vi "Process Messages.vi"(8 "error in (no error)":errorcluster, 11 "Mixer in":refnum<class "Mixer.lvclass">) -> (0 "error out":errorcluster, 3 "Mixer out":refnum<class "Mixer.lvclass">)   [LabVIEW 2019, in "Mixer.lvclass"]
uses:
  Mixer.lvclass
  Mixer.lvclass/Mixer.ctl
  Channel/Channel.lvclass
  Libraries/Messaging/Messaging.lvlib
  Libraries/Audio Processing/Audio Processing.lvlib
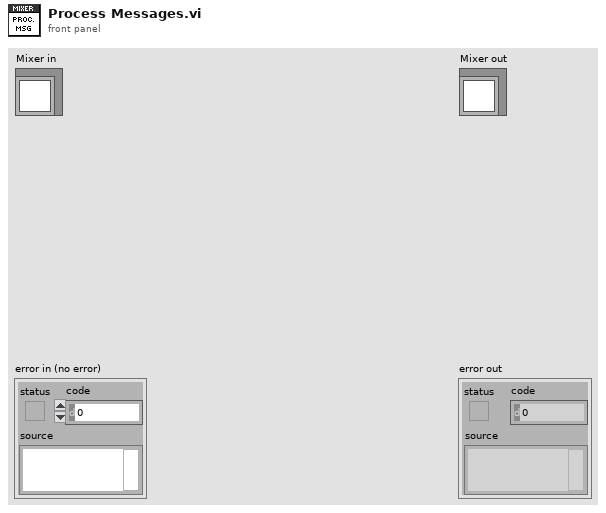
[diagram p1: front panel]
types:
  T1 = typedef "Messaging.lvlib/Message Cluster.ctl" = cluster{"Event":string, "Source":string, "Target":string, "Data":variant}
  T2 = typedef "Audio Processing.lvlib/Value Properties.ctl" = cluster{"Lower":dbl, "Upper":dbl}
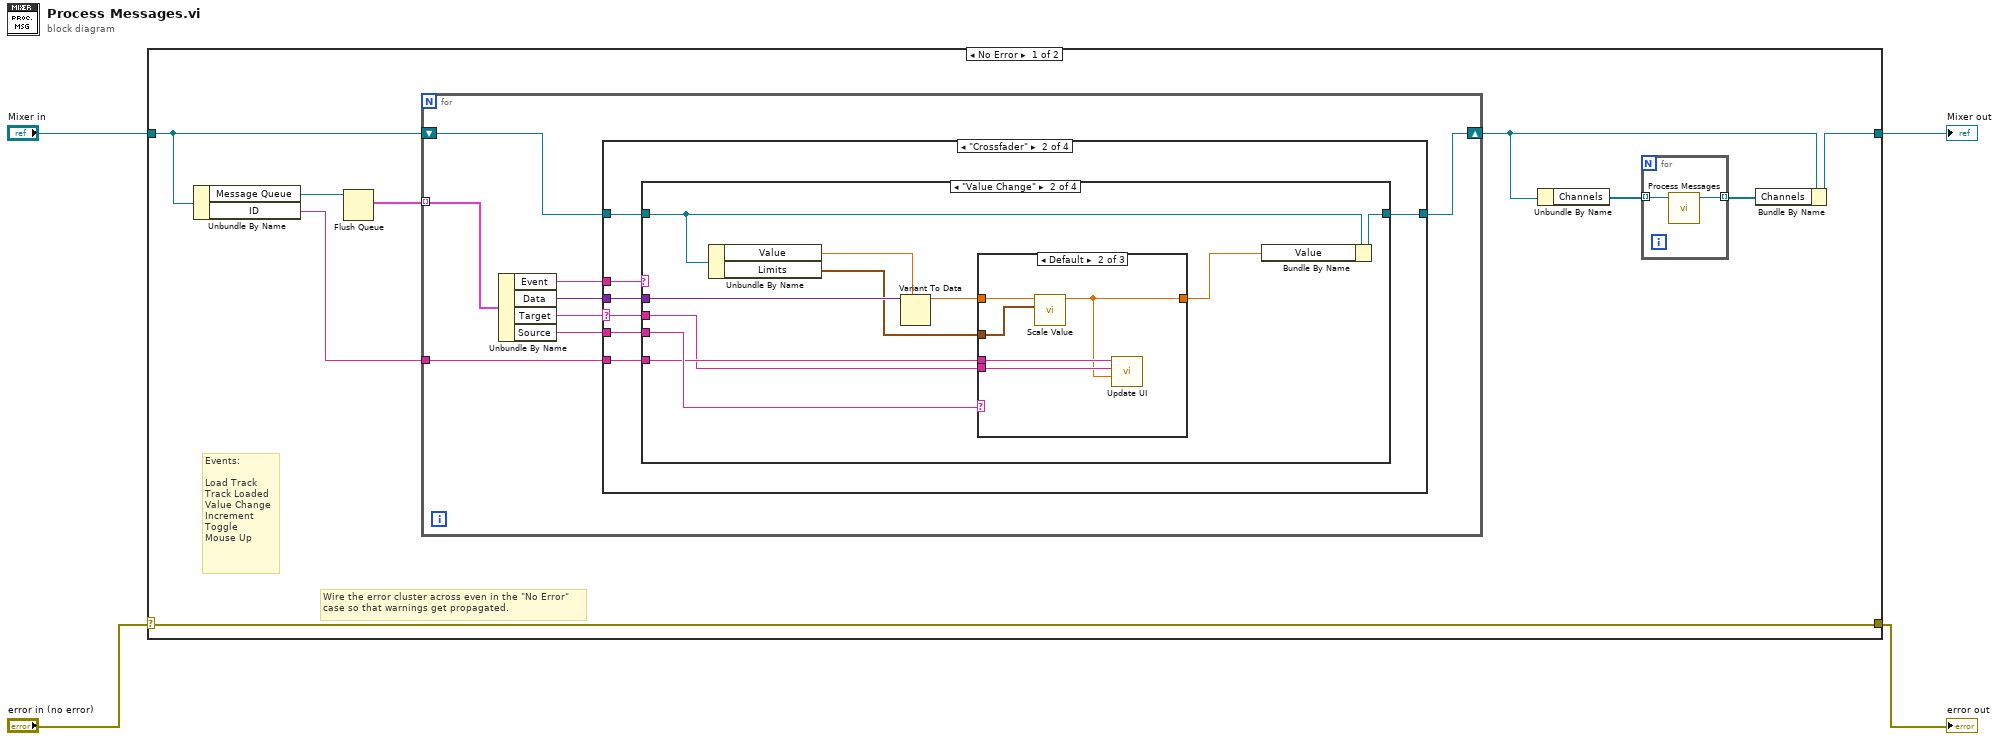
[diagram p0: block diagram]
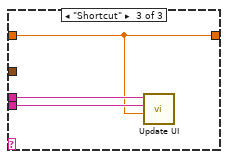
[diagram p5: hidden frame]
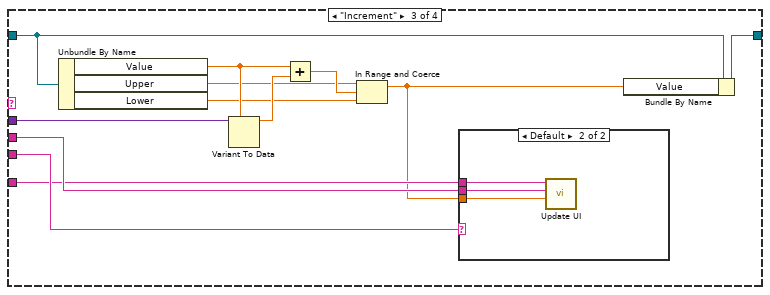
[diagram p6: hidden frame]
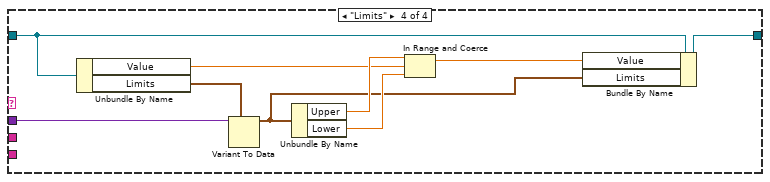
[diagram p8: hidden frame]
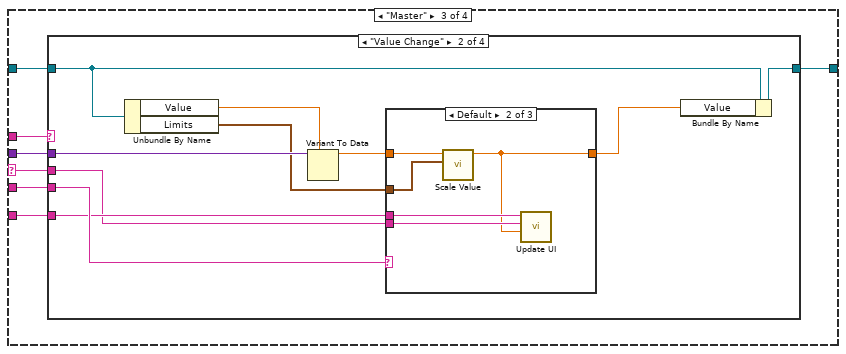
[diagram p9: hidden frame]
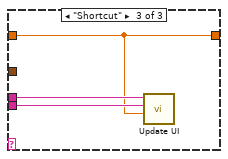
[diagram p12: hidden frame]
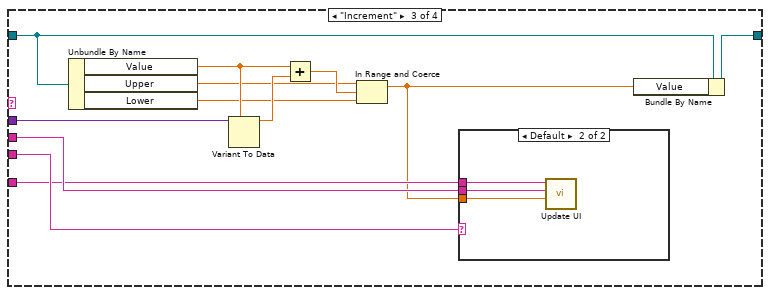
[diagram p13: hidden frame]
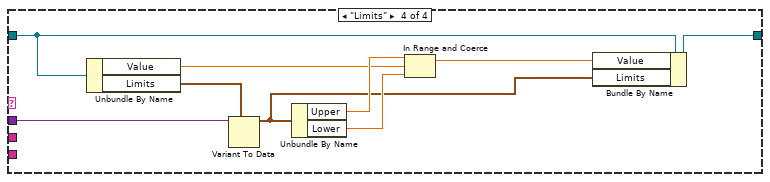
[diagram p15: hidden frame]
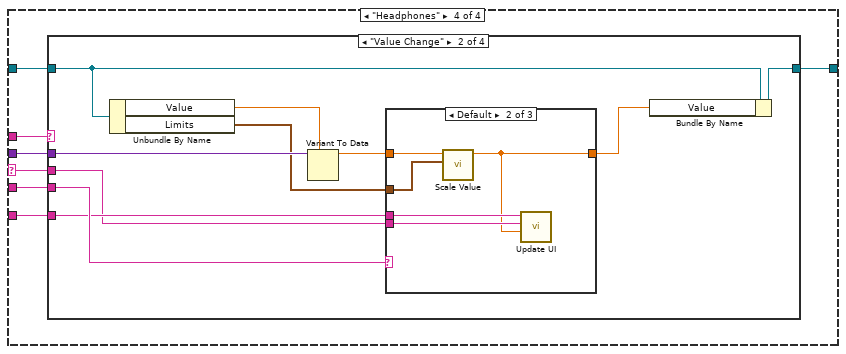
[diagram p16: hidden frame]
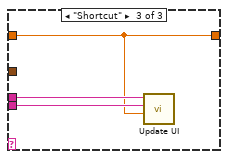
[diagram p19: hidden frame]
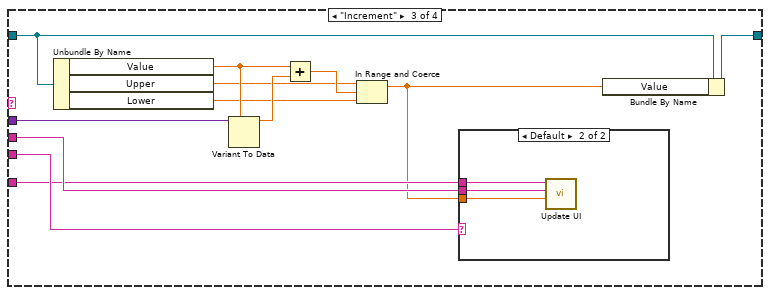
[diagram p20: hidden frame]
diagram:
  n1 = case shown="No Error" "error in (no error)" {
    selector: "error in (no error)" -> [w13 w179]
    tunnel: [w13 w179] -> w2
    tunnel: [w8 w178] -> w1
    tunnel: "Mixer in" -> [w12 w178]
    frame No Error {
      # "Events:\n\nLoad Track\nTrack Loaded\nValue Change\nIncrement\nToggle\nMouse Up"
      # "Wire the error cluster across even in the \"No Error\"\ncase so that warnings get propagated."
      n2 = Unbundle By Name(w12) -> ("Message Queue"=w7:refnum<queue>, "ID"=w5:string)
      n3 = Flush Queue(queue=w7) -> (remaining elements=w6:T1[])  [unwired: 1 in, 2 out]
      n4 = for {
        shift-right: [w22] -> w9
        shift-left: w12 -> [w23]
        tunnel: w6 -> [w21] mode=indexing
        tunnel: w5 -> [w16]
        n5 = Unbundle By Name(w21) -> ("Event"=w18:string, "Data"=w19:variant, "Target"=w20:string, "Source"=w17:string)
        n6 = case shown="\"Crossfader\"" w20 {
          selector: w20 -> [_ w26 w79 w130]
          tunnel: w23 -> [w24 w29 w82 w133]
          tunnel: [w24 w30 w76 w127] -> w22
          tunnel: w19 -> [_ w28 w80 w131]
          tunnel: w18 -> [_ w31 w81 w132]
          tunnel: w17 -> [_ w27 w78 w129]
          tunnel: w16 -> [_ w25 w77 w128]
          frame Default {
          }
          frame "Crossfader" {
            n7 = case shown="\"Value Change\"" w31 {
              tunnel: [w32 w39 w61 w73] -> w30
              tunnel: w29 -> [w32 w40 w62 w74]
              tunnel: w28 -> [_ w41 w63 w75]
              tunnel: w27 -> [_ w37 w60 _]
              tunnel: w26 -> [_ w35 w59 _]
              tunnel: w25 -> [_ w36 w58 _]
              frame Default {
              }
              frame "Value Change" {
                n8 = Unbundle By Name(w40) -> ("Value"=w42:dbl, "Limits"=w33:T2)
                n9 = Variant To Data(type=w42, Variant=w41) -> (data=w38:dbl)  [unwired: 1 in, 1 out]
                n10 = case shown="Default" w37 {
                  tunnel: w38 -> [w43 w46 w49]
                  tunnel: w35 -> [_ w48 w51]
                  tunnel: w36 -> [_ w47 w50]
                  tunnel: [w43 w44 w49] -> w34
                  tunnel: w33 -> [_ w45 _]
                  frame "UI" {
                  }
                  frame Default {
                    n11 = call "Scale Value.vi"("Limits"=w45, "Value"=w46) -> ("Scaled Value"=w44:dbl)  [unwired: 9 in]
                    n12 = call "Update UI.vi"("Data"=w44, "Target"=w48, "ID"=w47) -> ()  [unwired: 8 in, 1 out]
                  }
                  frame "Shortcut" {
                    n13 = call "Update UI.vi"("Data"=w49, "Target"=w51, "ID"=w50) -> ()  [unwired: 8 in, 1 out]
                  }
                }
                n14 = Bundle By Name(cluster=w40, "Value"=w34) -> (w39:refnum<class "Mixer.lvclass">)
              }
              frame "Increment" {
                n15 = Unbundle By Name(w62) -> ("Value"=w57:dbl, "Upper"=w54:dbl, "Lower"=w53:dbl)
                n16 = Variant To Data(type=w57, Variant=w63) -> (data=w56:dbl)  [unwired: 1 in, 1 out]
                n17 = Add(x=w57, y=w56) -> (x+y=w55:dbl)
                n18 = In Range and Coerce(upper limit=w54, x=w55, lower limit=w53) -> (coerced(x)=w52:dbl)  [unwired: 1 out]
                n19 = case shown="Default" w60 {
                  tunnel: w52 -> [_ w66]
                  tunnel: w59 -> [_ w65]
                  tunnel: w58 -> [_ w64]
                  frame "UI" {
                  }
                  frame Default {
                    n20 = call "Update UI.vi"("Data"=w66, "Target"=w65, "ID"=w64) -> ()  [unwired: 8 in, 1 out]
                  }
                }
                n21 = Bundle By Name(cluster=w62, "Value"=w52) -> (w61:refnum<class "Mixer.lvclass">)
              }
              frame "Limits" {
                n22 = Unbundle By Name(w74) -> ("Value"=w69:dbl, "Limits"=w67:T2)
                n23 = Variant To Data(type=w67, Variant=w75) -> (data=w68:T2)  [unwired: 1 in, 1 out]
                n24 = Unbundle By Name(w68) -> ("Upper"=w71:dbl, "Lower"=w70:dbl)
                n25 = In Range and Coerce(upper limit=w71, x=w69, lower limit=w70) -> (coerced(x)=w72:dbl)  [unwired: 1 out]
                n26 = Bundle By Name(cluster=w74, "Value"=w72, "Limits"=w68) -> (w73:refnum<class "Mixer.lvclass">)
              }
            }
          }
          frame "Master" {
            n27 = case shown="\"Value Change\"" w81 {
              tunnel: [w83 w90 w112 w124] -> w76
              tunnel: w82 -> [w83 w91 w113 w125]
              tunnel: w80 -> [_ w92 w114 w126]
              tunnel: w78 -> [_ w88 w111 _]
              tunnel: w79 -> [_ w86 w110 _]
              tunnel: w77 -> [_ w87 w109 _]
              frame Default {
              }
              frame "Value Change" {
                n28 = Unbundle By Name(w91) -> ("Value"=w93:dbl, "Limits"=w84:T2)
                n29 = Variant To Data(type=w93, Variant=w92) -> (data=w89:dbl)  [unwired: 1 in, 1 out]
                n30 = case shown="Default" w88 {
                  tunnel: w89 -> [w94 w97 w100]
                  tunnel: w86 -> [_ w99 w102]
                  tunnel: w87 -> [_ w98 w101]
                  tunnel: [w94 w95 w100] -> w85
                  tunnel: w84 -> [_ w96 _]
                  frame "UI" {
                  }
                  frame Default {
                    n31 = call "Scale Value.vi"("Limits"=w96, "Value"=w97) -> ("Scaled Value"=w95:dbl)  [unwired: 9 in]
                    n32 = call "Update UI.vi"("Data"=w95, "Target"=w99, "ID"=w98) -> ()  [unwired: 8 in, 1 out]
                  }
                  frame "Shortcut" {
                    n33 = call "Update UI.vi"("Data"=w100, "Target"=w102, "ID"=w101) -> ()  [unwired: 8 in, 1 out]
                  }
                }
                n34 = Bundle By Name(cluster=w91, "Value"=w85) -> (w90:refnum<class "Mixer.lvclass">)
              }
              frame "Increment" {
                n35 = Unbundle By Name(w113) -> ("Value"=w108:dbl, "Upper"=w105:dbl, "Lower"=w104:dbl)
                n36 = Variant To Data(type=w108, Variant=w114) -> (data=w107:dbl)  [unwired: 1 in, 1 out]
                n37 = Add(x=w108, y=w107) -> (x+y=w106:dbl)
                n38 = In Range and Coerce(upper limit=w105, x=w106, lower limit=w104) -> (coerced(x)=w103:dbl)  [unwired: 1 out]
                n39 = case shown="Default" w111 {
                  tunnel: w103 -> [_ w117]
                  tunnel: w110 -> [_ w116]
                  tunnel: w109 -> [_ w115]
                  frame "UI" {
                  }
                  frame Default {
                    n40 = call "Update UI.vi"("Data"=w117, "Target"=w116, "ID"=w115) -> ()  [unwired: 8 in, 1 out]
                  }
                }
                n41 = Bundle By Name(cluster=w113, "Value"=w103) -> (w112:refnum<class "Mixer.lvclass">)
              }
              frame "Limits" {
                n42 = Unbundle By Name(w125) -> ("Value"=w120:dbl, "Limits"=w118:T2)
                n43 = Variant To Data(type=w118, Variant=w126) -> (data=w119:T2)  [unwired: 1 in, 1 out]
                n44 = Unbundle By Name(w119) -> ("Upper"=w122:dbl, "Lower"=w121:dbl)
                n45 = In Range and Coerce(upper limit=w122, x=w120, lower limit=w121) -> (coerced(x)=w123:dbl)  [unwired: 1 out]
                n46 = Bundle By Name(cluster=w125, "Value"=w123, "Limits"=w119) -> (w124:refnum<class "Mixer.lvclass">)
              }
            }
          }
          frame "Headphones" {
            n47 = case shown="\"Value Change\"" w132 {
              tunnel: [w134 w141 w163 w175] -> w127
              tunnel: w133 -> [w134 w142 w164 w176]
              tunnel: w131 -> [_ w143 w165 w177]
              tunnel: w129 -> [_ w139 w162 _]
              tunnel: w130 -> [_ w137 w161 _]
              tunnel: w128 -> [_ w138 w160 _]
              frame Default {
              }
              frame "Value Change" {
                n48 = Unbundle By Name(w142) -> ("Value"=w144:dbl, "Limits"=w135:T2)
                n49 = Variant To Data(type=w144, Variant=w143) -> (data=w140:dbl)  [unwired: 1 in, 1 out]
                n50 = case shown="Default" w139 {
                  tunnel: w140 -> [w145 w148 w151]
                  tunnel: w137 -> [_ w150 w153]
                  tunnel: w138 -> [_ w149 w152]
                  tunnel: [w145 w146 w151] -> w136
                  tunnel: w135 -> [_ w147 _]
                  frame "UI" {
                  }
                  frame Default {
                    n51 = call "Scale Value.vi"("Limits"=w147, "Value"=w148) -> ("Scaled Value"=w146:dbl)  [unwired: 9 in]
                    n52 = call "Update UI.vi"("Data"=w146, "Target"=w150, "ID"=w149) -> ()  [unwired: 8 in, 1 out]
                  }
                  frame "Shortcut" {
                    n53 = call "Update UI.vi"("Data"=w151, "Target"=w153, "ID"=w152) -> ()  [unwired: 8 in, 1 out]
                  }
                }
                n54 = Bundle By Name(cluster=w142, "Value"=w136) -> (w141:refnum<class "Mixer.lvclass">)
              }
              frame "Increment" {
                n55 = Unbundle By Name(w164) -> ("Value"=w159:dbl, "Upper"=w156:dbl, "Lower"=w155:dbl)
                n56 = Variant To Data(type=w159, Variant=w165) -> (data=w158:dbl)  [unwired: 1 in, 1 out]
                n57 = Add(x=w159, y=w158) -> (x+y=w157:dbl)
                n58 = In Range and Coerce(upper limit=w156, x=w157, lower limit=w155) -> (coerced(x)=w154:dbl)  [unwired: 1 out]
                n59 = case shown="Default" w162 {
                  tunnel: w154 -> [_ w168]
                  tunnel: w161 -> [_ w167]
                  tunnel: w160 -> [_ w166]
                  frame "UI" {
                  }
                  frame Default {
                    n60 = call "Update UI.vi"("Data"=w168, "Target"=w167, "ID"=w166) -> ()  [unwired: 8 in, 1 out]
                  }
                }
                n61 = Bundle By Name(cluster=w164, "Value"=w154) -> (w163:refnum<class "Mixer.lvclass">)
              }
              frame "Limits" {
                n62 = Unbundle By Name(w176) -> ("Value"=w171:dbl, "Limits"=w169:T2)
                n63 = Variant To Data(type=w169, Variant=w177) -> (data=w170:T2)  [unwired: 1 in, 1 out]
                n64 = Unbundle By Name(w170) -> ("Upper"=w173:dbl, "Lower"=w172:dbl)
                n65 = In Range and Coerce(upper limit=w173, x=w171, lower limit=w172) -> (coerced(x)=w174:dbl)  [unwired: 1 out]
                n66 = Bundle By Name(cluster=w176, "Value"=w174, "Limits"=w170) -> (w175:refnum<class "Mixer.lvclass">)
              }
            }
          }
        }
      }
      n67 = Unbundle By Name(w9) -> ("Channels"=w11:refnum<class "Channel.lvclass">[])
      n68 = for {
        tunnel: w11 -> [w15] mode=indexing
        tunnel: [w14] -> w10 mode=indexing
        n69 = call "Process Messages.vi"("Channel in"=w15) -> ("Channel out"=w14:refnum<class "Channel.lvclass">)  [unwired: 9 in, 1 out]
      }
      n70 = Bundle By Name(cluster=w9, "Channels"=w10) -> (w8:refnum<class "Mixer.lvclass">)
    }
    frame Error {
    }
  }
  "error out" <- w2
  "Mixer out" <- w1
